vi "TextToVariant.vi"(7 "Data Type":variant, 8 "error in (no error)":errorcluster, 10 "Serializable Text":string, 11 "BlueTOMLSerializer in":refnum<class "BlueTOMLSerializer.lvclass">) -> (0 "error out":errorcluster, 2 "Variant out":variant, 3 "BlueTOMLSerializer out":refnum<class "BlueTOMLSerializer.lvclass">)   [LabVIEW 2019, in "BlueTOMLSerializer.lvlib" / "BlueTOMLSerializer.lvclass"]
uses:
  BlueTOMLSerializer.lvclass
  C:/Program Files (x86)/National Instruments/LabVIEW 2019/user.lib/Blue Origin/BlueSerialization/BlueSerializer/BlueSerializer.lvclass
  BlueTOMLSerializer.lvlib
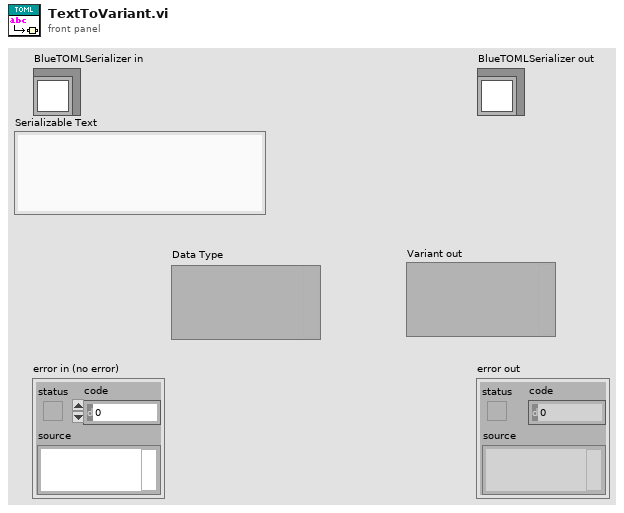
[diagram p1: front panel]
types:
  T1 = typedef "BlueTOMLSerializer.lvlib/TOML Value.ctl" = cluster{"\\type":enum16{"Table", "Array", "String", "Integer", "Float", "Boolean", "Offset Date-Time", "Local Date-Time", "Local Date", "Local Time"}, "ÿýÿýÿýÿýÿýÿþÿýÿýÿý%LV-TOML.lvlib:TOML Key-Value Pair.ctlÿýÿýÿýÿýÿýÿþÿýÿýÿýLV-TOML.lvlib:TOML Value.ctl$":variant}
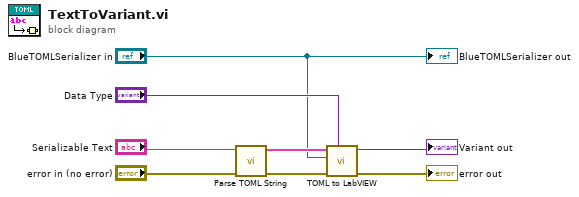
[diagram p0: block diagram]
diagram:
  n1 = call "Parse TOML String.vi"("error in (no error)"="error in (no error)", "String"="Serializable Text") -> ("error out"=w7:errorcluster, "Value"=w8:T1)  [unwired: 8 in]
  n2 = call "TOML to LabVIEW.vi"("Default Value"="Data Type", "error in (no error)"=w7, "BlueSerializer in"="BlueTOMLSerializer in", "TOML Value"=w8) -> ("error out"=→"error out":errorcluster, "LV Value"=→"Variant out":variant)  [unwired: 6 in]
  "BlueTOMLSerializer out" <- "BlueTOMLSerializer in"
